vi "Radio Get Received Energy.vi"(0 "a_data":dbl[](array[numeric]), 1 "a_inttime":dbl, 5 "a_startwav":dbl, 7 "a_endwav":dbl, 9 "a_surfacecm2":dbl, 11 "error in (no error)":errorcluster) -> (4 "a_data out":dbl[](array[numeric]), 6 "function return":i16, 14 "a_integral out":dbl, 15 "error out":errorcluster)   [LabVIEW 2013, in "AVSirrad.lvlib"]
doc: "DLL_API short int __stdcall Radio_GetReceivedEnergy\n(\n DataType *a_data,\n double a_startwav,\n double a_endwav,\n double a_surfacecm2,\n double a_inttime,\n double *a_integral\n);"
uses:
  AVSirrad.lvlib
  AVSIRRAD/Examples/Labview/build/AVSirrad.dll
panel:
  in  "a_integral":dbl
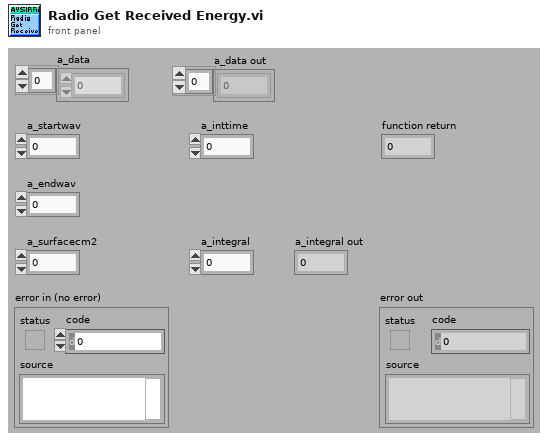
[diagram p1: front panel]
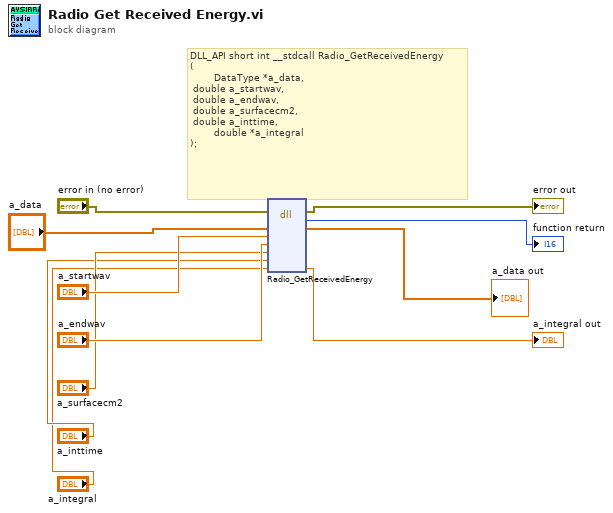
[diagram p0: block diagram]
diagram:
  # "DLL_API short int __stdcall Radio_GetReceivedEnergy\n(\n        DataType *a_data,\n\tdouble a_startwav,\n\tdouble a_endwav,\n\tdouble a_surfacecm2,\n\tdouble a_inttime,\n        double *a_integral\n);"
  n1 = dll-call lib="C:/AVSIRRAD/Examples/Labview/build/AVSirrad.*" fn="Radio_GetReceivedEnergy"(error in="error in (no error)", "a_data"="a_data", "a_startwav"="a_startwav", "a_endwav"="a_endwav", "a_surfacecm2"="a_surfacecm2", "a_inttime"="a_inttime", "a_integral"="a_integral") -> (error out=→"error out":errorcluster, "return type"=→"function return":i16, "a_data"=→"a_data out":dbl[], "a_integral"=→"a_integral out":dbl)  [unwired: 6 in, 1 out]
